vi "parse.vi"(8 "error in (no error)":errorcluster, 10 "Message":u8[](array[numeric]) format="%02x", 11 "T7Inclinometer in":refnum<class "T7Inclinometer.lvclass">) -> (0 "error out":errorcluster, 2 "Error":bool, 3 "T7Inclinometer out":refnum<class "T7Inclinometer.lvclass">)   [LabVIEW 2016, in "RTT7Inclinometer.lvlib" / "T7Inclinometer.lvclass"]
uses:
  T7Inclinometer.lvclass
  Common_RT_Utilities/U8ArrayParser/U8ArrayParserManualIndexing.lvclass
  T7Inclinometer.lvclass/T7Inclinometer.ctl
  DataTypes/T7InclinometerErrors.ctl
  Common_RT_Modbus/CRC/CRC.lvclass
  RTT7Inclinometer.lvlib
  Common_RT_Timestamp/Timestamp/Timestamp.lvclass
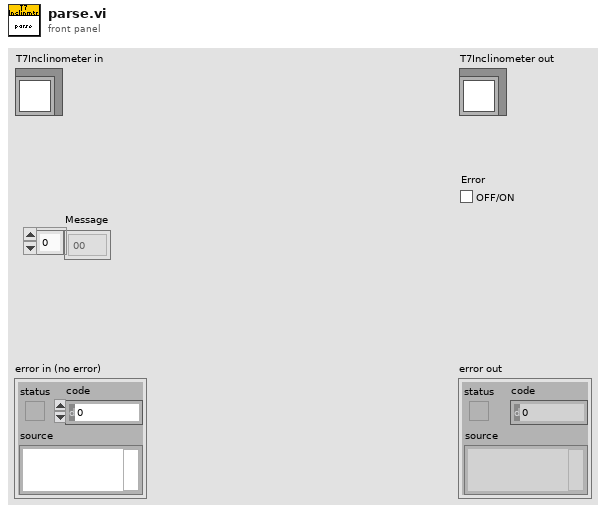
[diagram p1: front panel]
types:
  T1 = typedef "RTT7Inclinometer.lvlib/T7InclinometerErrors.ctl" = enum16{"None", "InvalidFunctionCodeError", "InvalidRegisterAddressError", "InvalidCRCError", "UnknownAddressError", "UnknownFunctionError", "InvalidResponseLengthError", "UnknownError"}
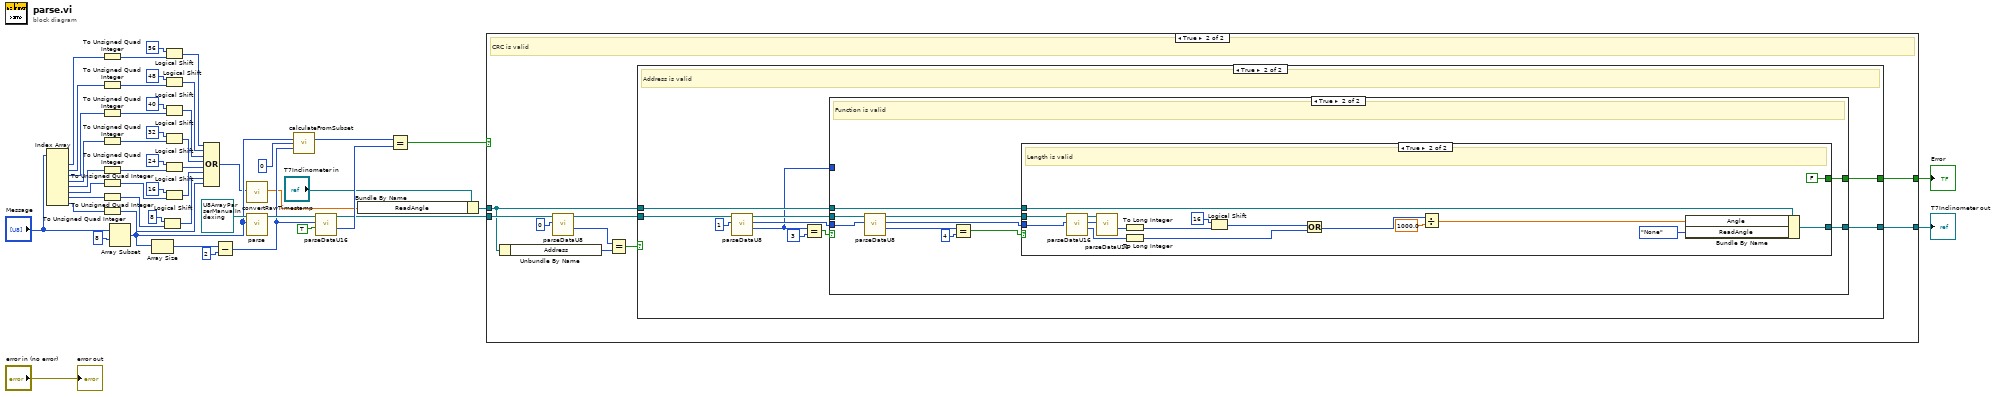
[diagram p0: block diagram]
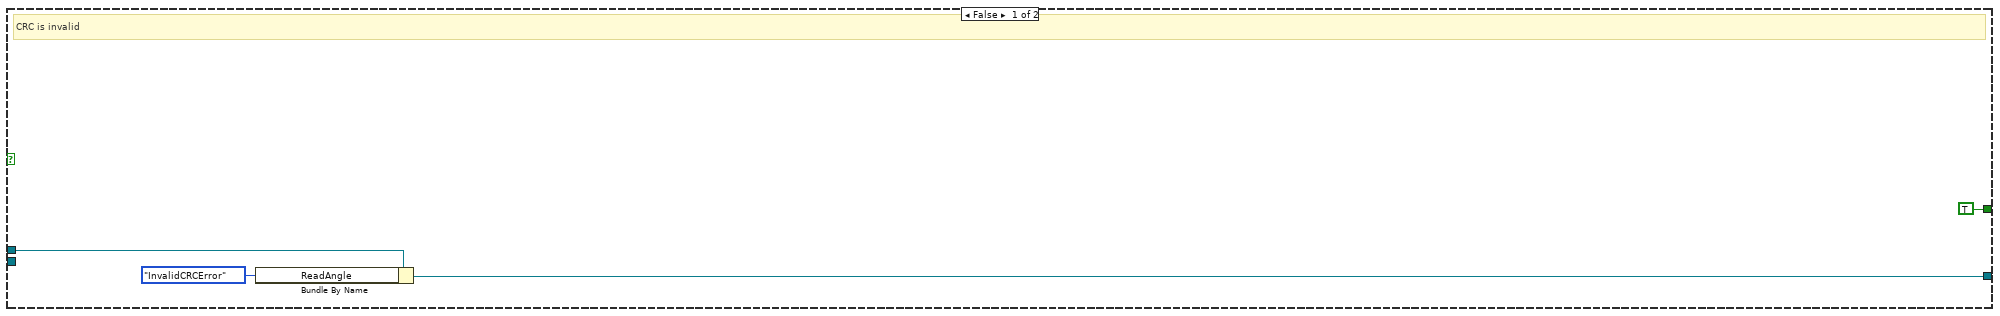
[diagram p2: hidden frame]
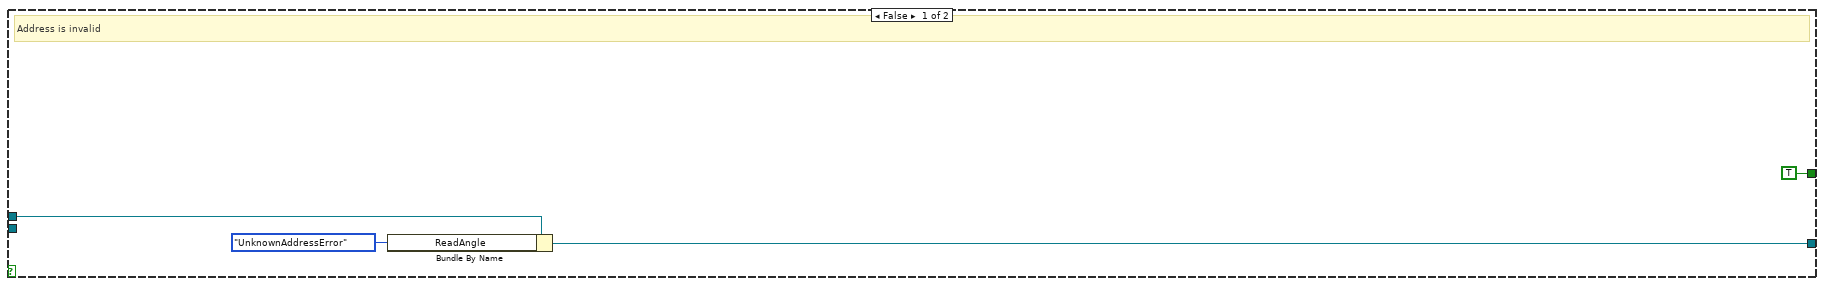
[diagram p3: hidden frame]
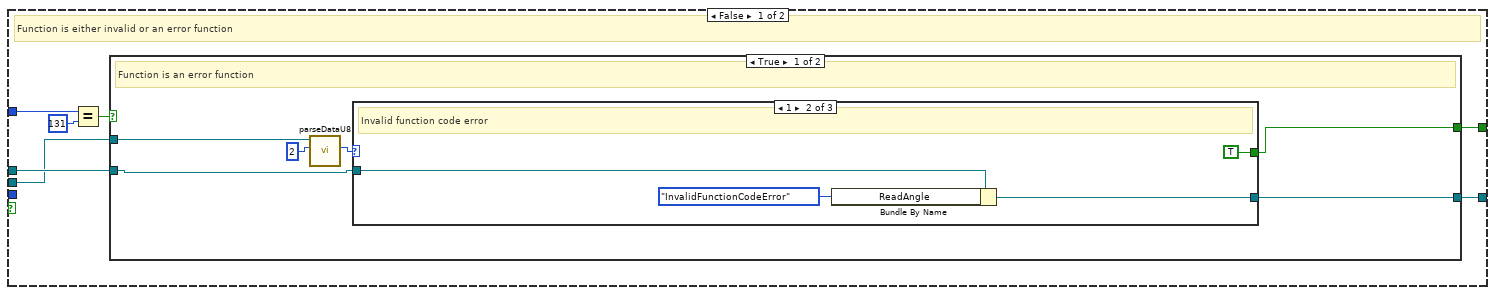
[diagram p4: hidden frame]
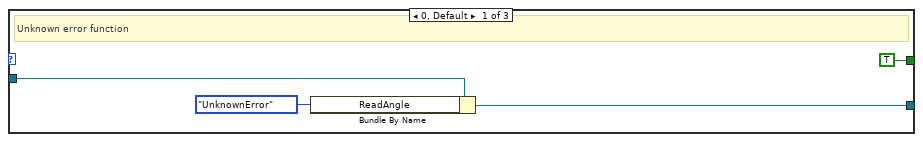
[diagram p5: hidden frame]
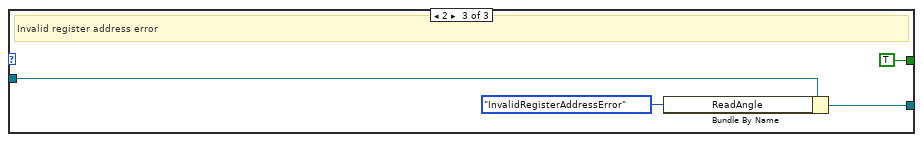
[diagram p6: hidden frame]
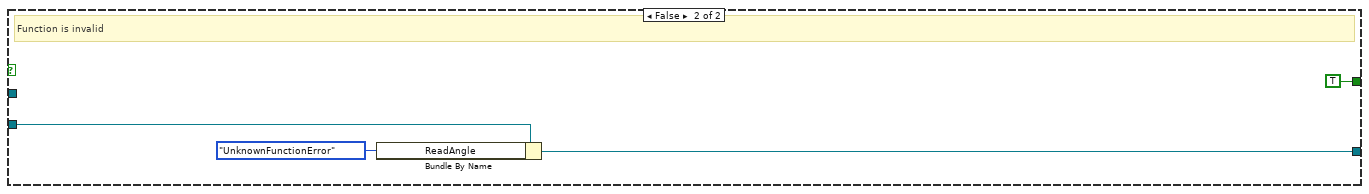
[diagram p7: hidden frame]
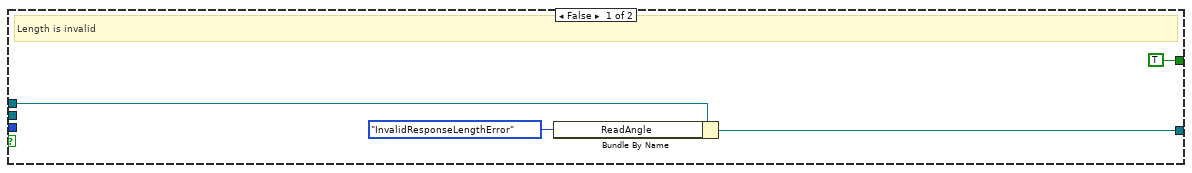
[diagram p8: hidden frame]
diagram:
  n1 = Index Array(array="Message") -> (element #1=w34:u8, element #2=w33:u8, element #3=w32:u8, element #4=w31:u8, element #5=w30:u8, element #6=w29:u8, element #7=w28:u8, element #8=w27:u8)  [unwired: 8 in]
  n2 = To Unsigned Quad Integer(1:w34) -> (0:w26:u64)
  n3 = To Unsigned Quad Integer(1:w33) -> (0:w25:u64)
  n4 = To Unsigned Quad Integer(1:w32) -> (0:w24:u64)
  n5 = To Unsigned Quad Integer(1:w31) -> (0:w23:u64)
  n6 = To Unsigned Quad Integer(1:w30) -> (0:w22:u64)
  n7 = To Unsigned Quad Integer(1:w29) -> (0:w21:u64)
  n8 = To Unsigned Quad Integer(1:w28) -> (0:w20:u64)
  n9 = To Unsigned Quad Integer(1:w27) -> (0:w5:u64)
  n10 = Array Subset(array="Message", index=8) -> (w35:u8[])  [unwired: 1 in]
  n11 = Array Size(array=w35) -> (size(s)=w48:i32)
  n12 = Logical Shift(y=i16 8, x=w20) -> (x << y=w6:u64)
  n13 = Logical Shift(y=i16 56, x=w26) -> (x << y=w12:u64)
  n14 = Logical Shift(y=i16 48, x=w25) -> (x << y=w11:u64)
  n15 = Logical Shift(y=i16 40, x=w24) -> (x << y=w10:u64)
  n16 = Logical Shift(y=i16 32, x=w23) -> (x << y=w9:u64)
  n17 = Logical Shift(y=i16 24, x=w22) -> (x << y=w8:u64)
  n18 = Logical Shift(y=i16 16, x=w21) -> (x << y=w7:u64)
  n19 = Compound Arithmetic op=OR(w12, w11, w10, w9, w8, w7, w6, w5) -> (w4:u64)
  n20 = Subtract(x=w48, y=2) -> (x-y=w43:i32)
  n21 = call "convertRawTimestamp.vi"("RawTimestamp"=w4) -> ("Timestamp"=w1:dbl)  [unwired: 8 in, 2 out]
  n22 = call "parse.vi"("Data"=w35, "U8ArrayParserManualIndexing in"=refnum<class "U8ArrayParserManualIndexing.lvclass"> refnum ("RTUtilities.lvlib:U8ArrayParserManualIndexing.lvclass")) -> ("U8ArrayParserManualIndexing out"=w46:refnum<class "U8ArrayParserManualIndexing.lvclass">)  [unwired: 8 in, 1 out]
  n23 = call "calculateFromSubset.vi"("Data"=w35, "StartIndex"=0, "Length"=w43) -> ("CRC"=w44:u16)  [unwired: 10 in, 2 out]
  n24 = call "parseDataU16.vi"("OverrideSwapBytes"=TRUE, "Index"=w43, "U8ArrayParserManualIndexing in"=w46) -> ("Data"=w45:u16, "U8ArrayParserManualIndexing out"=w41:refnum<class "U8ArrayParserManualIndexing.lvclass">)  [unwired: 5 in, 2 out]
  n25 = Bundle By Name(cluster="T7Inclinometer in", "ReadAngle"=w1) -> (w2:refnum<class "T7Inclinometer.lvclass">)
  n26 = Equal?(x=w44, y=w45) -> (x = y?=w42:bool)
  n27 = case shown="True" w42 {
    tunnel: w2 -> [w55 w58]
    tunnel: w41 -> [_ w62]
    tunnel: [w54 w64] -> w39
    tunnel: [TRUE ("Data.Telemetry.InvalidResponseLengthError") w63] -> w38
    frame False {
      # "CRC is invalid"
      n28 = Bundle By Name(cluster=w55, "ReadAngle"=T7InclinometerErrors."InvalidCRCError" ("Data.Telemetry.Errors")) -> (w54:refnum<class "T7Inclinometer.lvclass">)
    }
    frame True {
      # "CRC is valid"
      n29 = Unbundle By Name(w58) -> ("Address"=w57:u8)
      n30 = call "parseDataU8.vi"("Index"=0, "U8ArrayParserManualIndexing in"=w62) -> ("Data"=w59:u8, "U8ArrayParserManualIndexing out"=w61:refnum<class "U8ArrayParserManualIndexing.lvclass">)  [unwired: 6 in, 2 out]
      n31 = Equal?(x=w59, y=w57) -> (x = y?=w56:bool)
      n32 = case shown="True" w56 {
        tunnel: [w67 w74] -> w64
        tunnel: [TRUE ("Data.Telemetry.InvalidResponseLengthError") w73] -> w63
        tunnel: w61 -> [_ w72]
        tunnel: w58 -> [w68 w71]
        frame False {
          # "Address is invalid"
          n33 = Bundle By Name(cluster=w68, "ReadAngle"=T7InclinometerErrors."UnknownAddressError" ("Data.Telemetry.Errors")) -> (w67:refnum<class "T7Inclinometer.lvclass">)
        }
        frame True {
          # "Address is valid"
          n34 = call "parseDataU8.vi"("Index"=1, "U8ArrayParserManualIndexing in"=w72) -> ("Data"=w70:u8, "Index out"=w76:i32, "U8ArrayParserManualIndexing out"=w75:refnum<class "U8ArrayParserManualIndexing.lvclass">)  [unwired: 6 in, 1 out]
          n35 = Equal?(x=w70, y=u8 3) -> (x = y?=w77:bool)
          n36 = case shown="True" w77 {
            tunnel: w76 -> [_ w116]
            tunnel: w75 -> [w79 w117]
            tunnel: w71 -> [w85 w110]
            tunnel: [w84 w109] -> w74
            tunnel: [w83 w108] -> w73
            tunnel: w70 -> [w81 _]
            frame False {
              # "Function is either invalid or an error function"
              n37 = Equal?(x=w81, y=u8 131) -> (x = y?=w82:bool)
              n38 = case shown="True" w82 {
                tunnel: w85 -> [w87 w107]
                tunnel: [w88 w106] -> w84
                tunnel: [w86 TRUE ("Data.Telemetry.InvalidResponseLengthError")] -> w83
                tunnel: w79 -> [w91 _]
                frame True {
                  # "Function is an error function"
                  n39 = call "parseDataU8.vi"("Index"=2, "U8ArrayParserManualIndexing in"=w91) -> ("Index out"=w89:i32)  [unwired: 6 in, 3 out]
                  n40 = case shown="1" w89 {
                    tunnel: [w94 w98 w102] -> w88
                    tunnel: w87 -> [w95 w99 w103]
                    tunnel: [TRUE ("Data.Telemetry.UnknownError") TRUE ("Data.Telemetry.UnknownError") TRUE ("Data.Telemetry.UnknownError")] -> w86
                    frame 0, Default {
                      # "Unknown error function"
                      n41 = Bundle By Name(cluster=w95, "ReadAngle"=T7InclinometerErrors."UnknownError" ("Data.Telemetry.Errors")) -> (w94:refnum<class "T7Inclinometer.lvclass">)
                    }
                    frame 1 {
                      # "Invalid function code error"
                      n42 = Bundle By Name(cluster=w99, "ReadAngle"=T7InclinometerErrors."InvalidFunctionCodeError" ("Data.Telemetry.Errors")) -> (w98:refnum<class "T7Inclinometer.lvclass">)
                    }
                    frame 2 {
                      # "Invalid register address error"
                      n43 = Bundle By Name(cluster=w103, "ReadAngle"=T7InclinometerErrors."InvalidRegisterAddressError" ("Data.Telemetry.Errors")) -> (w102:refnum<class "T7Inclinometer.lvclass">)
                    }
                  }
                }
                frame False {
                  # "Function is invalid"
                  n44 = Bundle By Name(cluster=w107, "ReadAngle"=T7InclinometerErrors."UnknownFunctionError" ("Data.Telemetry.Errors")) -> (w106:refnum<class "T7Inclinometer.lvclass">)
                }
              }
            }
            frame True {
              # "Function is valid"
              n45 = call "parseDataU8.vi"("Index"=w116, "U8ArrayParserManualIndexing in"=w117) -> ("Data"=w115:u8, "Index out"=w112:i32, "U8ArrayParserManualIndexing out"=w111:refnum<class "U8ArrayParserManualIndexing.lvclass">)  [unwired: 6 in, 1 out]
              n46 = Equal?(x=w115, y=u8 4) -> (x = y?=w113:bool)
              n47 = case shown="True" w113 {
                tunnel: w112 -> [_ w137]
                tunnel: w111 -> [_ w138]
                tunnel: w110 -> [w121 w126]
                tunnel: [w120 w125] -> w109
                tunnel: [TRUE ("Data.Telemetry.InvalidResponseLengthError") FALSE ("Data.Telemetry.InvalidResponseLengthError")] -> w108
                frame False {
                  # "Length is invalid"
                  n48 = Bundle By Name(cluster=w121, "ReadAngle"=T7InclinometerErrors."InvalidResponseLengthError" ("Data.Telemetry.Errors")) -> (w120:refnum<class "T7Inclinometer.lvclass">)
                }
                frame True {
                  # "Length is valid"
                  n49 = call "parseDataU16.vi"("Index"=w137, "U8ArrayParserManualIndexing in"=w138) -> ("Data"=w131:u16, "Index out"=w136:i32, "U8ArrayParserManualIndexing out"=w135:refnum<class "U8ArrayParserManualIndexing.lvclass">)  [unwired: 6 in, 1 out]
                  n50 = call "parseDataU16.vi"("Index"=w136, "U8ArrayParserManualIndexing in"=w135) -> ("Data"=w134:u16)  [unwired: 6 in, 3 out]
                  n51 = To Long Integer(number=w134) -> (32bit integer=w133:i32)
                  n52 = To Long Integer(number=w131) -> (32bit integer=w129:i32)
                  n53 = Logical Shift(y=i16 16, x=w133) -> (x << y=w130:i32)
                  n54 = Or(x=w130, y=w129) -> (x .or. y?=w128:i32)
                  n55 = Divide(x=w128, y=1000.0) -> (x/y=w124:dbl)
                  n56 = Bundle By Name(cluster=w126, "Angle"=w124, "ReadAngle"=T7InclinometerErrors."None" ("Data.Telemetry.Errors")) -> (w125:refnum<class "T7Inclinometer.lvclass">)
                }
              }
            }
          }
        }
      }
    }
  }
  "T7Inclinometer out" <- w39
  "Error" <- w38
  "error out" <- "error in (no error)"
